vi "CarWash.vi"() -> ()   [LabVIEW 2018]
uses:
  Position.ctl
  MessageQueueData.ctl
  Command.ctl
panel:
  out "Time Remaining":u32
  in  "Vehicle Position":T1
  out "Car Wash Indicators":T2
  in  "stop":bool
  in  "Purchase Selection":cluster{"Deluxe Wash":bool, "Economy Wash":bool}
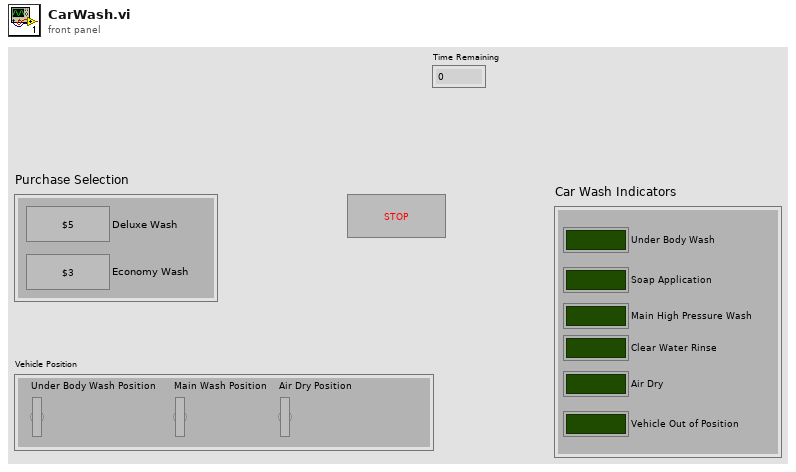
[diagram p1: front panel]
types:
  T1 = typedef "Position.ctl" = enum32{"Under Body Wash Position", "Main Wash Position", "Air Dry Position"}
  T2 = cluster{"Under Body Wash":bool, "Soap Application":bool, "Main High Pressure Wash":bool, "Clear Water Rinse":bool, "Air Dry":bool, "Vehicle Out of Position":bool}
  T3 = enum8{"Enabled", "Disabled", "Disabled and Grayed Out"}
  T4 = typedef "MessageQueueData.ctl" = cluster{"State":T5, "Data":variant}
  T5 = typedef "Command.ctl" = enum16{"Underbody Wash", "Soap Application", "Main High-Pressure Wash", "Clear Water Rinse", "Air Dry Cycle", "Stop"}
  T6 = cluster{"[0]":bool, "[1]":bool, "[2]":bool, "[3]":bool, "[4]":bool, "[5]":bool}
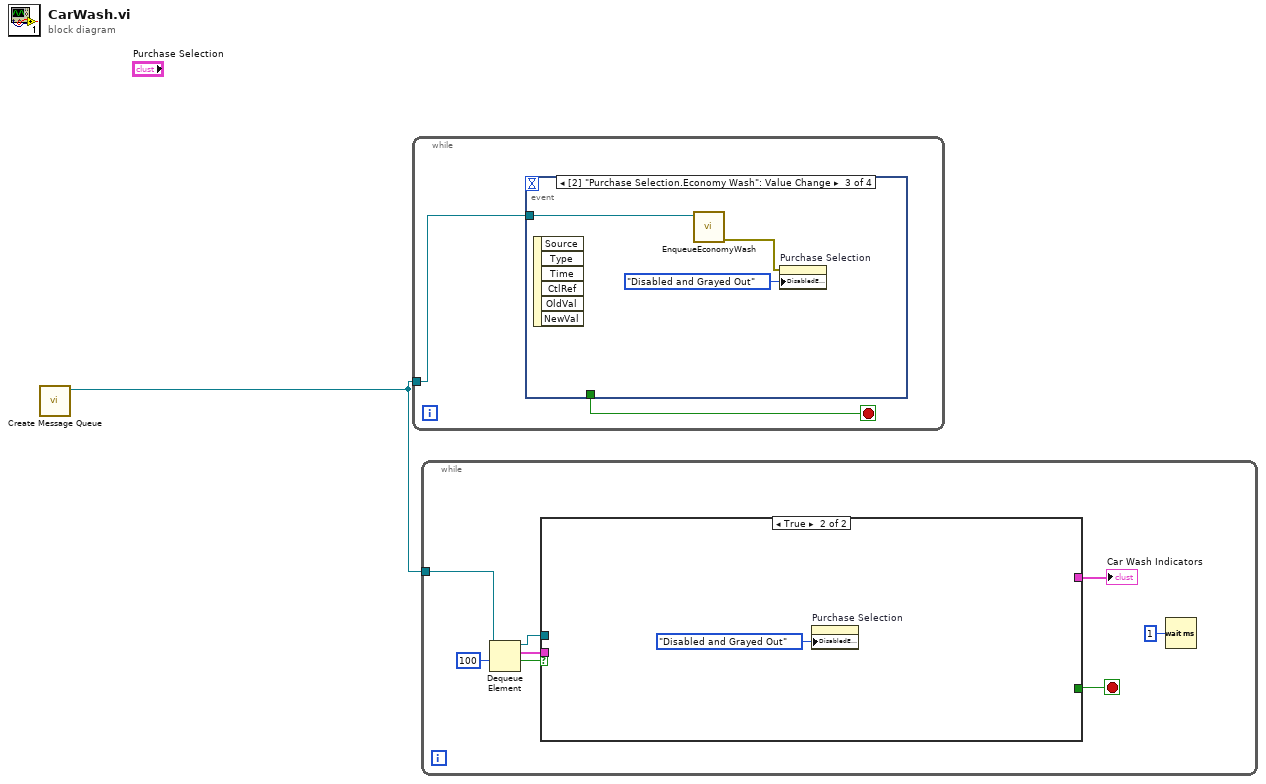
[diagram p0: block diagram]
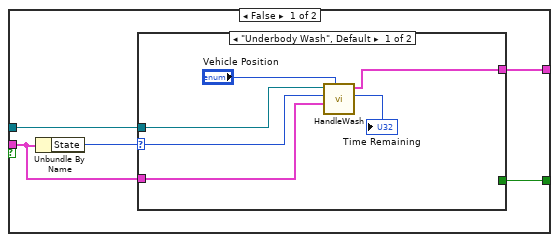
[diagram p2: hidden frame]
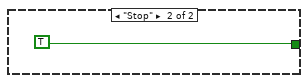
[diagram p3: hidden frame]
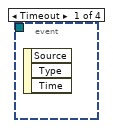
[diagram p4: hidden frame]
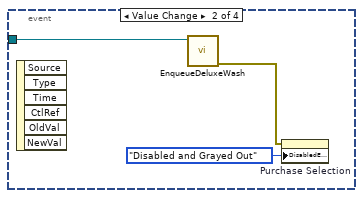
[diagram p5: hidden frame]
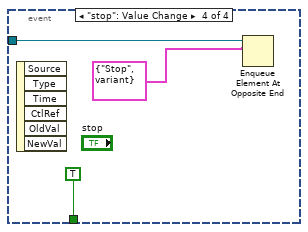
[diagram p6: hidden frame]
diagram:
  n1 = call "Create Message Queue.vi"() -> ("Queue out"=w1:refnum<queue>)  [unwired: 10 in, 1 out]
  n2 = while {
    tunnel: w1 -> [w2]
    stop <- w3 stop-if-true
    n3 = event shown="[2] \"Purchase Selection.Economy Wash\": Value Change" {
      selector: _ -> [_ _ _ _]
      dyn-events: _ -> [_ _ _ _]
      timeout: _ -> [_ _ _ _]
      tunnel: [_ _ _ TRUE ("NewVal")] -> w3
      tunnel: w2 -> [_ w6 w9 w11]
      event Timeout {
        n4 = event-data() -> ()  [unwired: 1 in, 3 out]
      }
      event "Purchase Selection.Deluxe Wash": Value Change {
        n5 = event-data() -> ()  [unwired: 1 in, 6 out]
        n6 = call "EnqueueDeluxeWash.vi"("Queue in"=w6) -> ("error out"=w4:errorcluster)  [unwired: 10 in]
        n7 = property on="Purchase Selection" class="Clust"(error in=w4, "DisabledEnum"=T3."Disabled and Grayed Out" ("Disabled")) -> ()  [unwired: 1 in, 2 out]
      }
      event "Purchase Selection.Economy Wash": Value Change {
        n8 = event-data() -> ()  [unwired: 1 in, 6 out]
        n9 = call "EnqueueEconomyWash.vi"("Queue in"=w9) -> ("error out"=w7:errorcluster)  [unwired: 9 in, 1 out]
        n10 = property on="Purchase Selection" class="Clust"(error in=w7, "DisabledEnum"=T3."Disabled and Grayed Out" ("Disabled")) -> ()  [unwired: 1 in, 2 out]
      }
      event "stop": Value Change {
        n11 = event-data() -> ()  [unwired: 1 in, 6 out]
        n12 = Enqueue Element At Opposite End(queue=w11, element=T4 {"State"=enum."Stop", "Data"=variant}) -> ()  [unwired: 2 in, 3 out]
      }
    }
  }
  n13 = while {
    tunnel: w1 -> [w20]
    stop <- w16 stop-if-true
    n14 = Dequeue Element(queue=w20, timeout in ms (-1)=100) -> (queue out=w15:refnum<queue>, element=w17:T4, timed out?=w19:bool)  [unwired: 1 in, 1 out]
    n15 = case shown="True" w19 {
      tunnel: w17 -> [w22 _]
      tunnel: [w24 _] -> w16
      tunnel: w15 -> [w23 _]
      tunnel: [w21 _] -> w14
      frame False {
        n16 = Unbundle By Name(w22) -> ("State"=w25:T5)
        n17 = case shown="\"Underbody Wash\", Default" w25 {
          selector: w25 -> [w27 _]
          tunnel: [_ TRUE] -> w24
          tunnel: w23 -> [w31 _]
          tunnel: w22 -> [w30 _]
          tunnel: [w26 _] -> w21
          frame "Underbody Wash", Default {
            n18 = call "HandleWash.vi"("Vehicle Position"="Vehicle Position", 9:w30, "Command"=w27, "queue in"=w31) -> ("Time Remaining"=→"Time Remaining":u32, "car wash indicators"=w26:T6)  [unwired: 6 in]
          }
          frame "Stop" {
          }
        }
      }
      frame True {
        n19 = property on="Purchase Selection" class="Clust"("DisabledEnum"=T3."Disabled and Grayed Out" ("Disabled")) -> ()  [unwired: 2 in, 2 out]
      }
    }
    "Car Wash Indicators" <- w14
    n20 = Wait (ms)(milliseconds to wait=u32 1) -> ()  [unwired: 1 out]
  }
